vi "test VIT Verify Person as JSON.vi"(8 "error in":errorcluster, 11 "Testing Approval Tests in":refnum<class "VITester Extension Tests.lvclass">) -> (0 "error out":errorcluster, 3 "Testing Approval Tests out":refnum<class "VITester Extension Tests.lvclass">)   [LabVIEW 2026, in "VITester Extension Tests.lvclass"]
uses:
  VITester Extension Tests.lvclass
  Common/Person/Person.lvclass
  Common/Person/Person.lvclass/Person.ctl
  Common/Person/Write First Name.vi
  Common/Person/Write Last Name.vi
  Common/Person/Write Title.vi
  VITester Extension Tests.lvclass/VITester Extension Tests.ctl
  Source/Extensions/VITester.Extension/VITester.Extension.lvlib
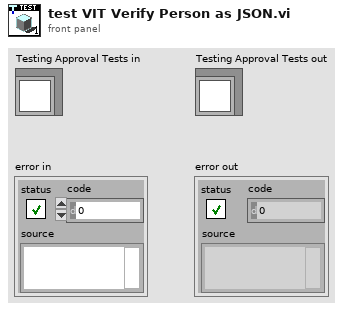
[diagram p1: front panel]
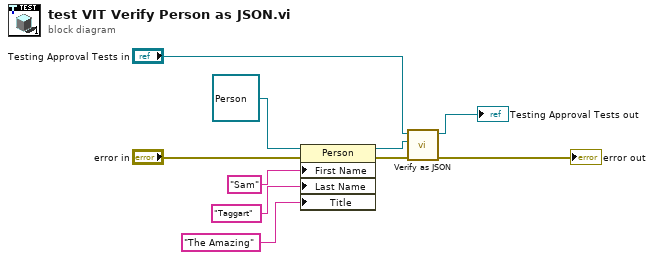
[diagram p0: block diagram]
diagram:
  n1 = property class="Person"(reference=refnum<class "Person.lvclass"> refnum ("Person.lvclass"), error in="error in", "First Name"="Sam", "Last Name"="Taggart", "Title"="The Amazing") -> (reference out=w1:refnum<class "Person.lvclass">, error out=w8:errorcluster)
  n2 = call "Verify as JSON.vi"("error in"=w8, "Anything"=w1, "TestCase in"="Testing Approval Tests in") -> ("error out"=→"error out":errorcluster, "TestCase out"=→"Testing Approval Tests out":refnum<class "VITester Extension Tests.lvclass">)  [unwired: 7 in]
